vi "411x_Create V Chans.vi"(5 "Device Ref in":T1 format="%.0x", 7 "# of V Channels to Add?":i16, 8 "error in":errorcluster, 9 "sense":T2=1008 caption="sense (out)" items=["Local"=1008, "Remote"=1009], 10 "Current Limit":dbl, 11 "Init Value":dbl) -> (0 "error out":errorcluster)   [LabVIEW 2023, in "NI PXIe-411x PS Custom Device.lvlib"]
uses:
  NI PXIe-411x PS Custom Device.lvlib
  <instrlib>/niDCPower/nidcpower.llb/niDCPower Sense.ctl
  <vilib>/NI VeriStand/Custom Device API/Custom Device Item Ref.ctl
  <vilib>/NI VeriStand/Custom Device API/Custom Device Channel.ctl
  <vilib>/NI VeriStand/Custom Device API/Custom Device Channel Type.ctl
  411x_Global.vi
  <vilib>/NI VeriStand/Custom Device API/Get Item Property (U16).vi
  <vilib>/NI VeriStand/Custom Device API/Get Item Property (Boolean).vi
  <vilib>/NI VeriStand/Custom Device API/Set Item Property (Double).vi
  <vilib>/NI VeriStand/Custom Device API/Set Item Property (U16).vi
  <vilib>/NI VeriStand/Custom Device API/Custom Device API.lvlib
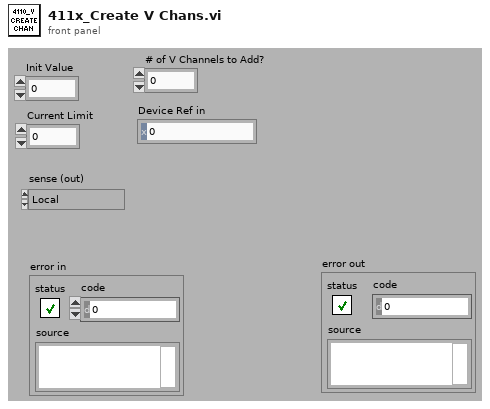
[diagram p1: front panel]
types:
  T1 = typedef "Custom Device API.lvlib/Custom Device Item Ref.ctl" = u64
  T2 = typedef "niDCPower Sense.ctl" = i32
  T3 = typedef "Custom Device API.lvlib/Custom Device Channel.ctl" = cluster{"Type":T4, "Units":string, "Default Value":dbl, "Faultable":bool, "Scalable":bool}
  T4 = typedef "Custom Device API.lvlib/Custom Device Channel Type.ctl" = enum16{"Input", "Output"}
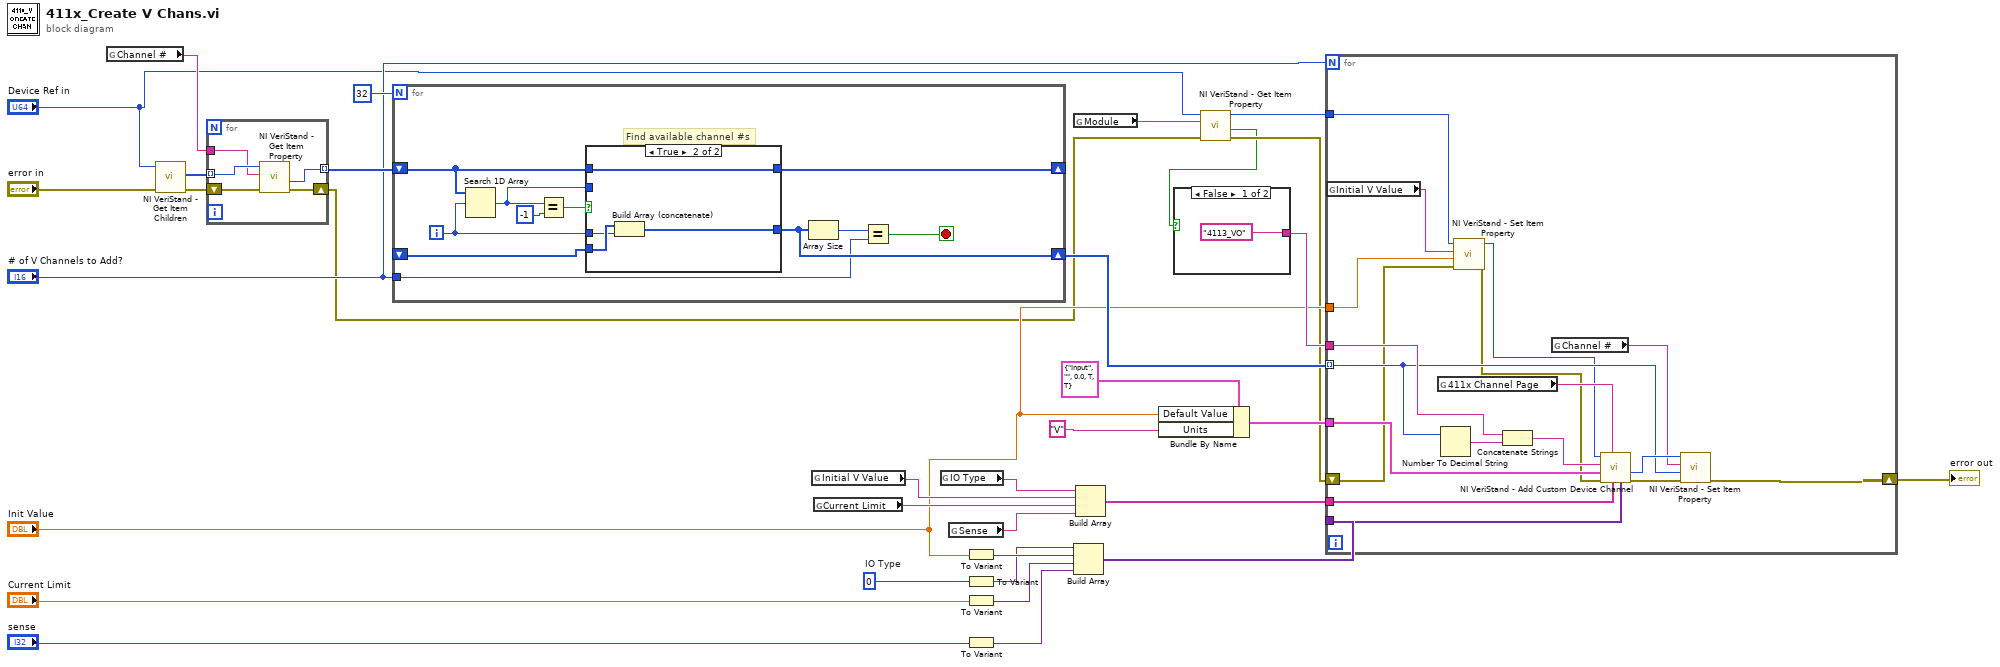
[diagram p0: block diagram]
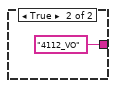
[diagram p2: hidden frame]
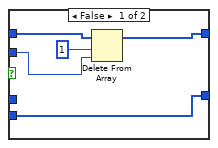
[diagram p3: hidden frame]
diagram:
  w11 = u16 0  # IO Type
  n1 = global read "411x_Global.vi" "Channel #"() -> (w16:string)
  n2 = call <vilib>:"NI VeriStand - Get Item Children.vi"("error in (no error)"="error in", "Item Ref in"="Device Ref in") -> ("error out"=w23:errorcluster, "Child Refs"=w24:T1[])  [unwired: 6 in, 2 out]
  n3 = for {
    tunnel: w24 -> [w38] mode=indexing
    shift-right: [w35] -> w3
    shift-left: w23 -> [w37]
    tunnel: w16 -> [w36]
    tunnel: [w34] -> w22 mode=indexing
    n4 = call-poly <vilib>:"NI VeriStand - Get Item Property.vi"("error in (no error)"=w37, "Property Name"=w36, "Item Ref in"=w38) -> ("error out"=w35:errorcluster, "Value"=w34:u16)  [unwired: 5 in, 2 out]
  }
  n5 = for {
    N: 32 -> [_]
    shift-right: [w42] -> w21
    shift-left: _ -> [w47]
    shift-right: [w43] -> _
    shift-left: w22 -> [w45]
    tunnel: "# of V Channels to Add?" -> [w40]
    i -> [w46]
    stop <- w39 stop-if-true
    # "Find available channel #s"
    n6 = Search 1D Array(1D array=w45, element=w46) -> (index of element=w44:i32)  [unwired: 1 in]
    n7 = Equal?(x=w44, y=-1) -> (x = y?=w48:bool)
    n8 = case shown="True" w48 {
      tunnel: w47 -> [w54 w58]
      tunnel: [w54 w57] -> w42
      tunnel: w46 -> [_ w56]
      tunnel: w45 -> [w53 w55]
      tunnel: w44 -> [w51 _]
      tunnel: [w50 w55] -> w43
      frame False {
        n9 = Delete From Array(array=w53, length=1, index=w51) -> (array with subset deleted=w50:u16[])  [unwired: 1 out]
      }
      frame True {
        n10 = Build Array (concatenate)(w58, w56) -> (w57:i32[])
      }
    }
    n11 = Array Size(array=w42) -> (size(s)=w41:i32)
    n12 = Equal?(x=w41, y=w40) -> (x = y?=w39:bool)
  }
  n13 = global read "411x_Global.vi" "Initial V Value"() -> (w14:string)
  n14 = global read "411x_Global.vi" "Current Limit"() -> (w13:string)
  n15 = global read "411x_Global.vi" "IO Type"() -> (w15:string)
  n16 = global read "411x_Global.vi" "Sense"() -> (w12:string)
  n17 = To Variant(anything="Init Value") -> (Variant=w29:variant)
  n18 = To Variant(anything=w11) -> (Variant=w28:variant)
  n19 = To Variant(anything="Current Limit") -> (Variant=w30:variant)
  n20 = To Variant(anything="sense") -> (Variant=w31:variant)
  n21 = global read "411x_Global.vi" "Module"() -> (w5:string)
  n22 = Build Array(w28, w29, w30, w31) -> (w32:variant[])
  n23 = Build Array(w15, w14, w13, w12) -> (w33:string[])
  n24 = Bundle By Name(cluster=T3 {"Type"=enum."Input", "Units"="", "Default Value"=0.0, "Faultable"=TRUE, "Scalable"=TRUE} ("Channel"), "Default Value"="Init Value", "Units"="V") -> (w19:T3)
  n25 = call-poly <vilib>:"NI VeriStand - Get Item Property.vi"("error in (no error)"=w3, "Property Name"=w5, "Item Ref in"="Device Ref in") -> ("error out"=w2:errorcluster, "Value"=w1:bool, "Item Ref out"=w4:T1)  [unwired: 5 in, 1 out]
  n26 = case shown="False" w1 {
    tunnel: ["4113_VO" "4112_VO"] -> w27
    frame False {
    }
    frame True {
    }
  }
  n27 = for {
    N: "# of V Channels to Add?" -> [_]
    shift-right: [w67] -> w26
    shift-left: w2 -> [w63]
    tunnel: w19 -> [w78]
    tunnel: w27 -> [w77]
    tunnel: w32 -> [w72]
    tunnel: w33 -> [w71]
    tunnel: w21 -> [w70] mode=indexing
    tunnel: "Init Value" -> [w64]
    tunnel: w4 -> [w61]
    n28 = global read "411x_Global.vi" "Initial V Value"() -> (w65:string)
    n29 = global read "411x_Global.vi" "411x Channel Page"() -> (w68:string)
    n30 = Number To Decimal String(number=w70) -> (decimal integer string=w76:string)  [unwired: 1 in]
    n31 = call-poly <vilib>:"NI VeriStand - Set Item Property.vi"("error in (no error)"=w63, "Value"=w64, "Property Name"=w65, "Item Ref in"=w61) -> ("error out"=w62:errorcluster, "Item Ref out"=w66:T1)  [unwired: 5 in, 1 out]
    n32 = Concatenate Strings(w77, w76) -> (w75:string)
    n33 = global read "411x_Global.vi" "Channel #"() -> (w69:string)
    n34 = call <vilib>:"NI VeriStand - Add Custom Device Channel.vi"("Property Values"=w72, "Property names"=w71, "GUID (Default Channel)"=w68, "error in (no error)"=w62, "Channel"=w78, "Channel Name"=w75, "Parent Ref in"=w66) -> ("error out"=w74:errorcluster, "Channel Ref"=w73:T1)  [unwired: 1 in, 2 out]
    n35 = call-poly <vilib>:"NI VeriStand - Set Item Property.vi"("error in (no error)"=w74, "Value"=w70, "Property Name"=w69, "Item Ref in"=w73) -> ("error out"=w67:errorcluster)  [unwired: 5 in, 2 out]
  }
  "error out" <- w26
